vi "Unpress Latching Boolean.vi"(11 "Ctl Refnum":refnum<vi>) -> ()   [LabVIEW 2015, in "ActorEvents.lvlib" / "ControlEventHandler.lvclass"]
uses:
  ControlEventHandler.lvclass
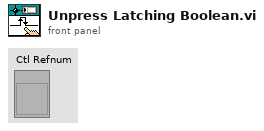
[diagram p1: front panel]
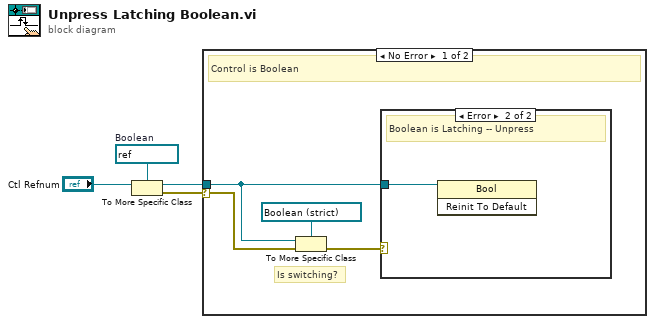
[diagram p0: block diagram]
diagram:
  w3 = refnum<vi> refnum  # Boolean
  n1 = To More Specific Class(target class=w3, reference="Ctl Refnum") -> (specific class reference=w1:refnum<vi>, error out=w2:errorcluster)  [unwired: 1 in]
  n2 = case shown="No Error" w2 {
    selector: w2 -> [w7 _]
    tunnel: w1 -> [w5 _]
    frame No Error {
      # "Is switching?"
      # "Control is Boolean"
      n3 = To More Specific Class(target class=refnum<vi> refnum ("Switching"), reference=w5, error in=w7) -> (error out=w6:errorcluster)  [unwired: 1 out]
      n4 = case shown="Error" w6 {
        tunnel: w5 -> [_ w9]
        frame No Error {
          # "Boolean is NOT latching -- Do nothing"
        }
        frame Error {
          # "Boolean is Latching -- Unpress"
          n5 = invoke class="Bool" method="Reinit To Default"(reference=w9) -> ()  [unwired: 2 in, 3 out]
        }
      }
    }
    frame Error {
      # "Not a Boolean"
    }
  }
